vi "ReadDoubleGlobals.vi"(8 "error in (no error)":errorcluster, 9 "variable count":i32, 10 "variable number":i32, 11 "controller in":refnum<k24>) -> (0 "error out":errorcluster, 2 "values":dbl[](array[numeric]), 3 "controller out":refnum<k24>)   [LabVIEW 2010]
uses:
  c:/aerotech/controller/5.xx.xxx/ensemble/pc/labview/2010/bin/Aerotech.Ensemble.dll
  bin/Aerotech.Ensemble.dll
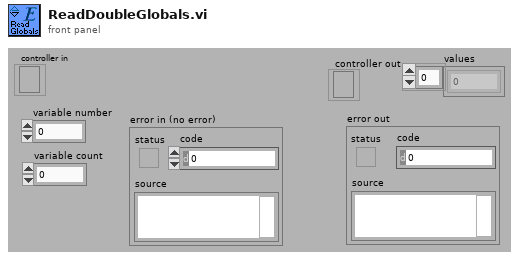
[diagram p1: front panel]
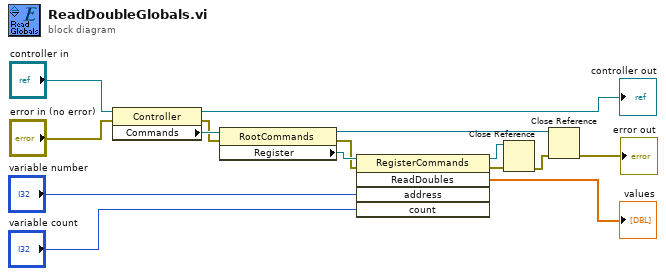
[diagram p0: block diagram]
diagram:
  n1 = property class="Controller"(reference="controller in", error in="error in (no error)") -> (reference out=→"controller out":refnum<k24>, error out=w12:errorcluster, "Commands"=w13:refnum<k24>)
  n2 = property class="RootCommands"(reference=w13, error in=w12) -> (reference out=w5:refnum<k24>, error out=w10:errorcluster, "Register"=w11:refnum<k24>)
  n3 = invoke class="RegisterCommands" method="ReadDoubles"(reference=w11, error in=w10, "address"="variable number", "count"="variable count") -> (reference out=w7:refnum<k24>, error out=w6:errorcluster, "ReadDoubles"=→"values":dbl[])  [unwired: 1 in, 2 out]
  n4 = Close Reference(reference=w7, error in (no error)=w6) -> (error out=w4:errorcluster)
  n5 = Close Reference(reference=w5, error in (no error)=w4) -> (error out=→"error out":errorcluster)
